vi "Ping1D (SubVi).vi"(8 "Comm. Delay":u32=500, 11 "Cluster":T1={"Connections"={"Ping1D - A"={"Connection"="", "error"={"status"=FALSE, "code"=0, "source"=""}, "Distance"=0.0, "FIFO"={"rt fifo"=refnum, "error"={"status"=FALSE, "code"=0, "source"=""}}}, "Ping1D - B"={"Connection"="", "error"={"status"=FALSE, "code"=0, "source"=""}, "Distance"=0.0, "FIFO"={"rt fifo"=refnum, "error"={"status"=FALSE, "code"=0, "source"=""}}}, "IMU"={"Error"={"status"=FALSE, "code"=0, "source"=""}, "FIFO"={"fifo"=refnum, "error"={"status"=FALSE, "code"=0, "source"=""}}}, "MotorControl"={"Rear"={"Error PWM"={"status"=FALSE, "code"=0, "source"=""}, "Error Direction"={"status"=FALSE, "code"=0, "source"=""}}, "Left"={"Error PWM"={"status"=FALSE, "code"=0, "source"=""}, "Error Direction"={"status"=FALSE, "code"=0, "source"=""}}, "Right"={"Error PWM"={"status"=FALSE, "code"=0, "source"=""}, "Error Direction"={"status"=FALSE, "code"=0, "source"=""}}}}, "sensorData"={"IMU Data"={"X-Axis"=0.0, "Y-Axis"=0.0, "Z-Axis"=0.0}}, "outputData"={"Rotation Angle"=0.0, "Rotation Vector"={"x"=0.0, "y"=0.0, "z"=0.0}, "PING A distance"=0.0, "Ping B distance"=0.0, "angles"={"roll"=0.0, "pitch"=0.0, "yaw"=0.0}}, "Writer"={"endpoint"="", "error"={"status"=FALSE, "code"=0, "source"=""}}, "PID"={"reinitialize?"=FALSE, "Depth"={"setpoint"=0.0, "Gains"={"proportional gain (Kc)"=1.0, "integral time (Ti, min)"=0.01, "derivative time (Td, min)"=0.0}}, "Roll"={"setpoint"=0.0, "Gains"={"proportional gain (Kc)"=1.0, "integral time (Ti, min)"=0.01, "derivative time (Td, min)"=0.0}}}} {"PID"."Roll"."setpoint" format="%.2f"; "PID"."Roll"."Gains"."derivative time (Td, min)" format="%.3f"; "PID"."Roll"."Gains"."integral time (Ti, min)" format="%.3f"; "PID"."Roll"."Gains"."proportional gain (Kc)" format="%.3f"; "PID"."Depth"."setpoint" format="%.2f"; "PID"."Depth"."Gains"."derivative time (Td, min)" format="%.3f"; "PID"."Depth"."Gains"."integral time (Ti, min)" format="%.3f"; "PID"."Depth"."Gains"."proportional gain (Kc)" format="%.3f"}) -> (3 "Cluster out":T1={"Connections"={"Ping1D - A"={"Connection"="", "error"={"status"=FALSE, "code"=0, "source"=""}, "Distance"=0.0, "FIFO"={"rt fifo"=refnum, "error"={"status"=FALSE, "code"=0, "source"=""}}}, "Ping1D - B"={"Connection"="", "error"={"status"=FALSE, "code"=0, "source"=""}, "Distance"=0.0, "FIFO"={"rt fifo"=refnum, "error"={"status"=FALSE, "code"=0, "source"=""}}}, "IMU"={"Error"={"status"=FALSE, "code"=0, "source"=""}, "FIFO"={"fifo"=refnum, "error"={"status"=FALSE, "code"=0, "source"=""}}}, "MotorControl"={"Rear"={"Error PWM"={"status"=FALSE, "code"=0, "source"=""}, "Error Direction"={"status"=FALSE, "code"=0, "source"=""}}, "Left"={"Error PWM"={"status"=FALSE, "code"=0, "source"=""}, "Error Direction"={"status"=FALSE, "code"=0, "source"=""}}, "Right"={"Error PWM"={"status"=FALSE, "code"=0, "source"=""}, "Error Direction"={"status"=FALSE, "code"=0, "source"=""}}}}, "sensorData"={"IMU Data"={"X-Axis"=0.0, "Y-Axis"=0.0, "Z-Axis"=0.0}}, "outputData"={"Rotation Angle"=0.0, "Rotation Vector"={"x"=0.0, "y"=0.0, "z"=0.0}, "PING A distance"=0.0, "Ping B distance"=0.0, "angles"={"roll"=0.0, "pitch"=0.0, "yaw"=0.0}}, "Writer"={"endpoint"="", "error"={"status"=FALSE, "code"=0, "source"=""}}, "PID"={"reinitialize?"=FALSE, "Depth"={"setpoint"=0.0, "Gains"={"proportional gain (Kc)"=1.0, "integral time (Ti, min)"=0.01, "derivative time (Td, min)"=0.0}}, "Roll"={"setpoint"=0.0, "Gains"={"proportional gain (Kc)"=1.0, "integral time (Ti, min)"=0.01, "derivative time (Td, min)"=0.0}}}} {"PID"."Roll"."setpoint" format="%.2f"; "PID"."Roll"."Gains"."derivative time (Td, min)" format="%.3f"; "PID"."Roll"."Gains"."integral time (Ti, min)" format="%.3f"; "PID"."Roll"."Gains"."proportional gain (Kc)" format="%.3f"; "PID"."Depth"."setpoint" format="%.2f"; "PID"."Depth"."Gains"."derivative time (Td, min)" format="%.3f"; "PID"."Depth"."Gains"."integral time (Ti, min)" format="%.3f"; "PID"."Depth"."Gains"."proportional gain (Kc)" format="%.3f"})   [LabVIEW 2019]
uses:
  Connections.ctl
  ROVsensorData.ctl
  ROVdataOut.ctl
  ROVcluster.ctl
panel:
  out "Ping B response":string
  out "Ping A response":string
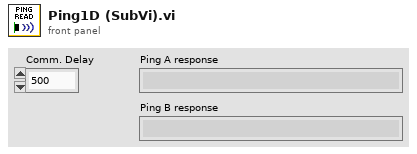
[diagram p1: front panel]
types:
  T1 = typedef "ROVcluster.ctl" = cluster{"Connections":T2, "sensorData":T3, "outputData":T4, "Writer":cluster{"endpoint":refnum<k21>, "error":errorcluster}, "PID":cluster{"reinitialize?":bool, "Depth":cluster{"setpoint":dbl, "Gains":cluster{"proportional gain (Kc)":dbl, "integral time (Ti, min)":dbl, "derivative time (Td, min)":dbl}}, "Roll":cluster{"setpoint":dbl, "Gains":cluster{"proportional gain (Kc)":dbl, "integral time (Ti, min)":dbl, "derivative time (Td, min)":dbl}}}}
  T2 = typedef "Connections.ctl" = cluster{"Ping1D - A":cluster{"Connection":refnum<visa-resource-name>, "error":errorcluster, "Distance":dbl, "FIFO":cluster{"rt fifo":refnum<k33>, "error":errorcluster}}, "Ping1D - B":cluster{"Connection":refnum<visa-resource-name>, "error":errorcluster, "Distance":dbl, "FIFO":cluster{"rt fifo":refnum<k33>, "error":errorcluster}}, "IMU":cluster{"Error":errorcluster, "FIFO":cluster{"fifo":refnum<k33>, "error":errorcluster}}, "MotorControl":cluster{"Rear":cluster{"Error PWM":errorcluster, "Error Direction":errorcluster}, "Left":cluster{"Error PWM":errorcluster, "Error Direction":errorcluster}, "Right":cluster{"Error PWM":errorcluster, "Error Direction":errorcluster}}}
  T3 = typedef "ROVsensorData.ctl" = cluster{"IMU Data":cluster{"X-Axis":dbl, "Y-Axis":dbl, "Z-Axis":dbl}}
  T4 = typedef "ROVdataOut.ctl" = cluster{"Rotation Angle":dbl, "Rotation Vector":cluster{"x":dbl, "y":dbl, "z":dbl}, "PING A distance":dbl, "Ping B distance":dbl, "angles":cluster{"roll":dbl, "pitch":dbl, "yaw":dbl}}
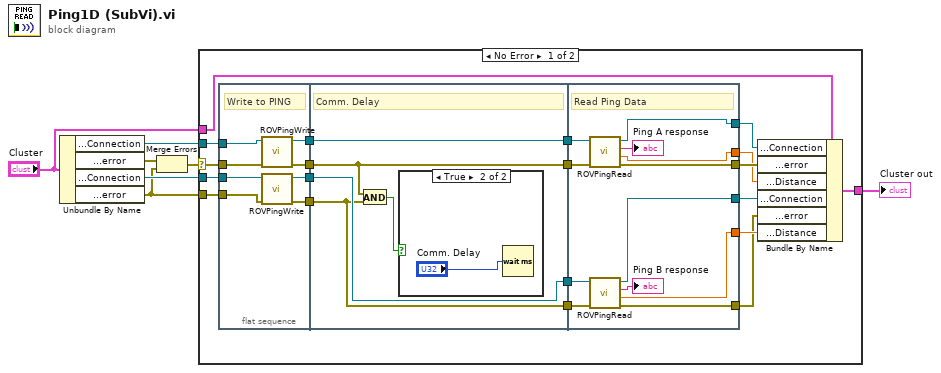
[diagram p0: block diagram]
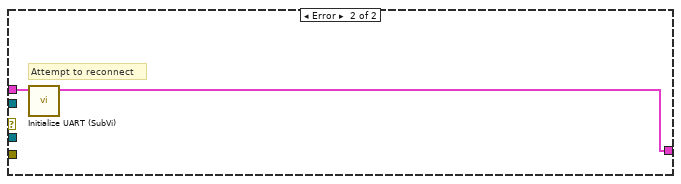
[diagram p3: hidden frame]
diagram:
  n1 = Unbundle By Name("Cluster") -> ("Connections.Ping1D - A.Connection"=w7:refnum<visa-resource-name>, "Connections.Ping1D - A.error"=w6:errorcluster, "Connections.Ping1D - B.Connection"=w3:refnum<visa-resource-name>, "Connections.Ping1D - B.error"=w1:errorcluster)
  n2 = Merge Errors(w6, w1) -> (w2:errorcluster)
  n3 = case shown="No Error" w2 {
    selector: w2 -> [w22 _]
    tunnel: w7 -> [w23 _]
    tunnel: "Cluster" -> [w21 w54]
    tunnel: [w20 w55] -> w4
    tunnel: w3 -> [w16 _]
    tunnel: w1 -> [w15 _]
    frame No Error {
      n4 = flat-sequence {
        tunnel: w22 -> [w35]
        tunnel: w23 -> [w34]
        tunnel: [w33] -> w27
        tunnel: [w32] -> w26
        tunnel: w16 -> [w31]
        tunnel: w15 -> [w30]
        tunnel: [w29] -> w13
        tunnel: [w28] -> w12
        tunnel: w27 -> [w40]
        tunnel: w26 -> [w38]
        tunnel: [w40] -> w25
        tunnel: [w38] -> w24
        tunnel: [w39] -> w14
        tunnel: w13 -> [w39]
        tunnel: w12 -> [w37]
        tunnel: [w37] -> w11
        tunnel: w25 -> [w52]
        tunnel: w24 -> [w53]
        tunnel: [w51] -> w19
        tunnel: [w50] -> w18
        tunnel: [w49] -> w17
        tunnel: w14 -> [w47]
        tunnel: w11 -> [w46]
        tunnel: [w45] -> w10
        tunnel: [w44] -> w9
        tunnel: [w43] -> w8
        frame #0 {
          # "Write to PING"
          n5 = call "ROVPingWrite.vi"("error in (no error)"=w35, "VISA Refnum in"=w34) -> ("error out"=w32:errorcluster, "VISA Refnum out"=w33:refnum<visa-resource-name>)  [unwired: 8 in]
          n6 = call "ROVPingWrite.vi"("error in (no error)"=w30, "VISA Refnum in"=w31) -> ("error out"=w28:errorcluster, "VISA Refnum out"=w29:refnum<visa-resource-name>)  [unwired: 8 in]
        }
        frame #1 {
          # "Comm. Delay"
          n7 = And(x=w38, y=w37) -> (x .and. y?=w36:bool)
          n8 = case shown="True" w36 {
            frame False {
              # "Skip in case\nof both returning\nerror"
            }
            frame True {
              n9 = Wait (ms)(milliseconds to wait="Comm. Delay") -> ()  [unwired: 1 out]
            }
          }
        }
        frame #2 {
          # "Read Ping Data"
          n10 = call "ROVPingRead.vi"("error in (no error)"=w53, "VISA Refnum in"=w52) -> ("error out"=w50:errorcluster, "Afstand Ping1D (m)"=w49:dbl, "Ping1d svar"=→"Ping A response":string, "VISA Refnum out"=w51:refnum<visa-resource-name>)  [unwired: 6 in]
          n11 = call "ROVPingRead.vi"("error in (no error)"=w46, "VISA Refnum in"=w47) -> ("error out"=w43:errorcluster, "Afstand Ping1D (m)"=w44:dbl, "Ping1d svar"=→"Ping B response":string, "VISA Refnum out"=w45:refnum<visa-resource-name>)  [unwired: 6 in]
        }
      }
      n12 = Bundle By Name(cluster=w21, "Connections.Ping1D - A.Connection"=w19, "Connections.Ping1D - A.error"=w18, "Connections.Ping1D - A.Distance"=w17, "Connections.Ping1D - B.Connection"=w10, "Connections.Ping1D - B.error"=w8, "Connections.Ping1D - B.Distance"=w9) -> (w20:T1)
    }
    frame Error {
      # "Attempt to reconnect"
      n13 = call "Initialize UART (SubVi).vi"("Cluster"=w54) -> ("Cluster out"=w55:T1)  [unwired: 10 in]
    }
  }
  "Cluster out" <- w4
